vi "USERTESTVI).vi"() -> (2 "buttin pressed":i32, 3 "布尔":bool)   [LabVIEW 2018]
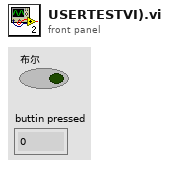
[diagram p1: front panel]
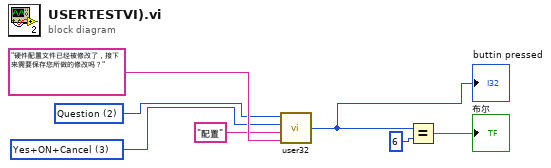
[diagram p0: block diagram]
diagram:
  w2 = u16 3 items=["OK", "OK+Cancel", "Abort+Retry+Ignore", "Yes+ON+Cancel", "Yes+No", "Retry+Cancel", "Cancel+Retry+Continue"] ("Buttons")
  w1 = u16 2 items=["None", "Critical", "Question", "Exclamation", "Infomation"] ("Icon")
  n1 = call "user32.vi"("Icon"=w1, "Buttons"=w2, "Ipcaption"="配置", "IP Text"="硬件配置文件已经被修改了，接下来需要保存您所做的修改吗？") -> ("buttin pressed"=w7:i32)  [unwired: 1 out]
  "buttin pressed" <- w7
  n2 = Equal?(x=w7, y=6) -> (x = y?=→"布尔":bool)
